vi "GetPWD.vi"(3 "error in (no error)":errorcluster caption="错误输入（无错误）", 4 "连接模式":enum16{"单机", "联网"}(ring), 5 "User_Name":string) -> (0 "error out":errorcluster caption="错误输出", 1 "Permission":string, 2 "Password":string)   [LabVIEW 2020]
uses:
  <vilib>/addons/database/Connection.llb/DB Tools Open Connec (String).vi
  <vilib>/addons/database/Connection.llb/Conn Execute.vi
  <vilib>/addons/database/Recordset.llb/Rec Fetch String Data (R).vi
  <vilib>/addons/database/Recordset.llb/Rec Destroy - Connection.vi
  <vilib>/addons/database/NI_Database_API.lvlib
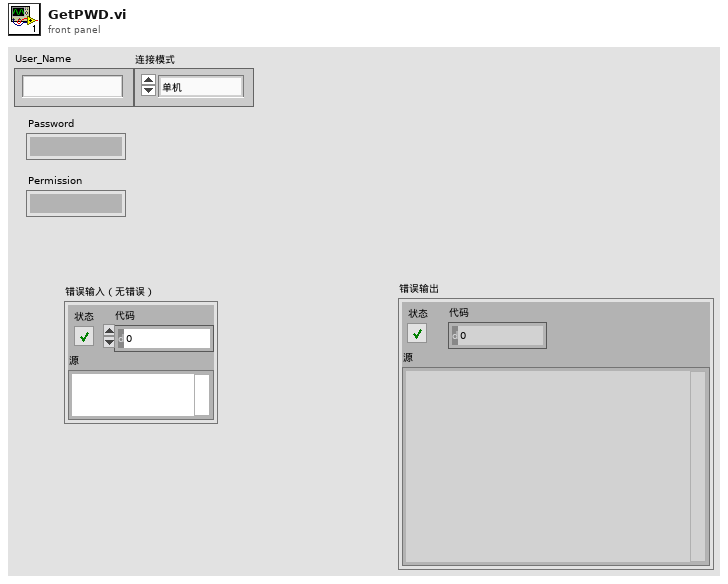
[diagram p1: front panel]
types:
  T1 = typedef "NI_Database_API.lvlib/Conn ObjectReference.ctl" = refnum<k1>
  T2 = typedef "NI_Database_API.lvlib/Rec ObjectReference.ctl" = refnum<k1>
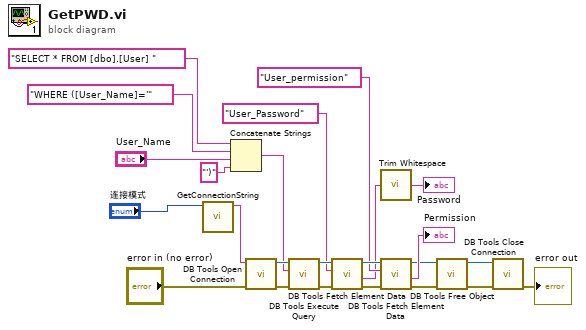
[diagram p0: block diagram]
diagram:
  n1 = call "GetConnectionString.vi"("连接模式"="连接模式") -> ("连接字符串"=w4:string)  [unwired: 5 in, 1 out]
  n2 = Concatenate Strings("SELECT * FROM [dbo].[User] " ("SQL query"), "WHERE ([User_Name]='", "User_Name", "')") -> (w18:string)
  n3 = call-poly <vilib>:"DB Tools Open Connection.vi"("error in (no error)"="error in (no error)", "connection information"=w4) -> ("error out"=w16:errorcluster, "connection reference"=w24:T1)  [unwired: 6 in]
  n4 = call-poly <vilib>:"DB Tools Execute Query.vi"("error in (no error)"=w16, "SQL query"=w18, "connection reference"=w24) -> ("error out"=w15:errorcluster, "recordset reference"=w23:T2)  [unwired: 5 in]
  n5 = call-poly <vilib>:"DB Tools Fetch Element Data.vi"("error in (no error)"=w15, "column index"="User_Password", "recordset reference"=w23) -> ("error out"=w14:errorcluster, "data"=w3:string, "recordset reference out"=w17:T2)  [unwired: 4 in]
  n6 = call <vilib>:"Trim Whitespace.vi"("string"=w3) -> ("trimmed string"=→"Password":string)  [unwired: 1 in]
  n7 = call-poly <vilib>:"DB Tools Fetch Element Data.vi"("error in (no error)"=w14, "column index"="User_permission", "recordset reference"=w17) -> ("error out"=w8:errorcluster, "data"=→"Permission":string, "recordset reference out"=w10:T2)  [unwired: 4 in]
  n8 = call-poly <vilib>:"DB Tools Free Object.vi"("error in (no error)"=w8, "recordset reference"=w10) -> ("error out"=w7:errorcluster, "connection reference"=w9:T1)  [unwired: 8 in]
  n9 = call <vilib>:"DB Tools Close Connection.vi"("error in (no error)"=w7, "connection reference"=w9) -> ("error out"=→"error out":errorcluster)  [unwired: 5 in]
